vi "MSScript_Format_IonGate.vi"(9 "ValueArray":string[](array[string]), 10 "TagArray":string[](array[string]), 11 "MSScript in":refnum<class "MSScript.lvclass">) -> (0 "ValueErrorArray":bool[](array[boolean]), 1 "TagErrorArray":bool[](array[boolean]), 2 "ParamErrorArray":bool[](array[boolean]), 3 "Data":variant, 4 "#ofParamError":bool)   [LabVIEW 2018, in "MSScript.lvclass"]
uses:
  MSScript.lvclass
  Ctl/MSEditorParam ionGate.ctl
  MSScript_Transform_Boolean.vi
  MSScript_Transform_Extended.vi
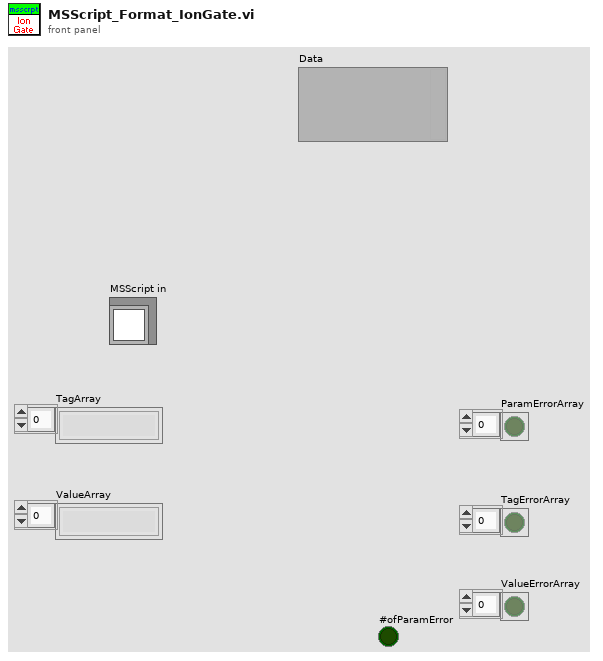
[diagram p1: front panel]
types:
  T1 = typedef "MSEditorParam ionGate.ctl" = cluster{"trialTime":ext, "TPH":ext, "enableAGC":bool}
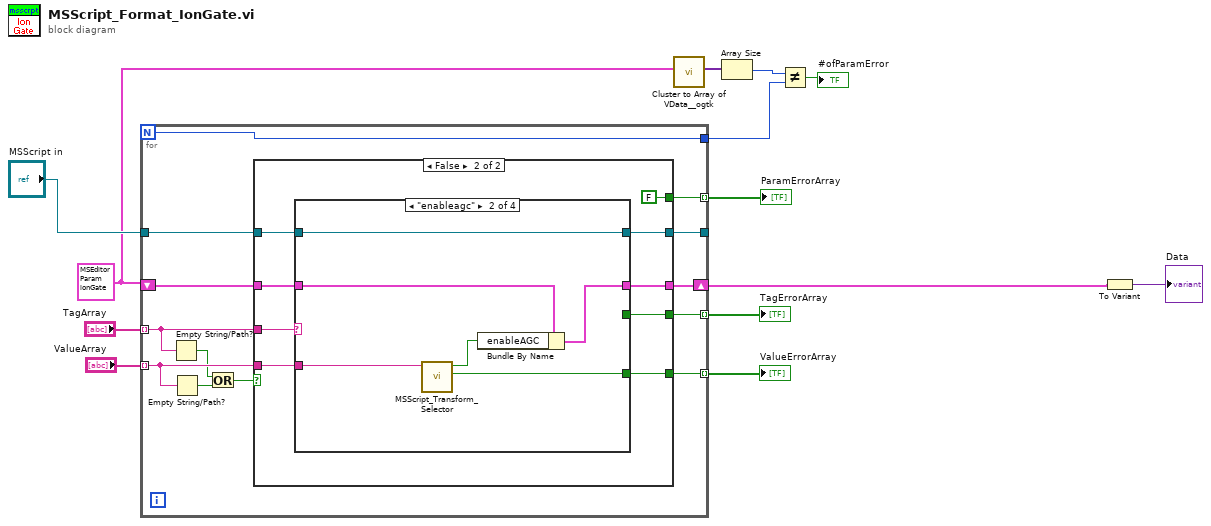
[diagram p0: block diagram]
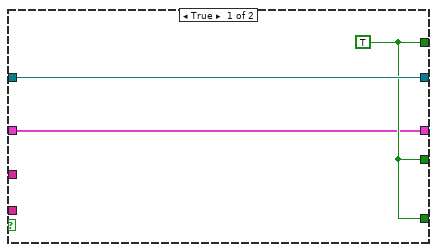
[diagram p2: hidden frame]
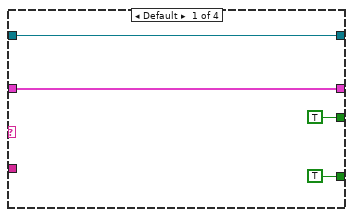
[diagram p3: hidden frame]
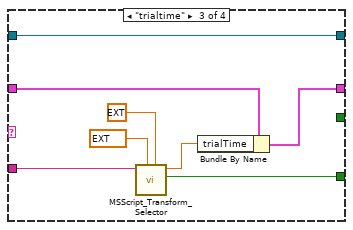
[diagram p4: hidden frame]
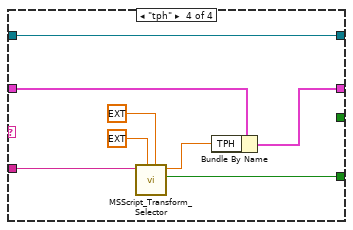
[diagram p5: hidden frame]
diagram:
  w4 = T1 {"trialTime"=0.1, "TPH"=1.0, "enableAGC"=FALSE} ("ParamValueType")
  n1 = for {
    N -> [w14]
    tunnel: "TagArray" -> [w22] mode=indexing
    tunnel: "ValueArray" -> [w21] mode=indexing
    tunnel: [w26] -> w11 mode=indexing
    tunnel: "MSScript in" -> [w25]
    tunnel: [w24] -> w10 mode=indexing
    tunnel: [w23] -> _
    tunnel: [w17] -> w9 mode=indexing
    shift-right: [w15] -> w2
    shift-left: w4 -> [w16]
    tunnel: [w14] -> w3
    n2 = Empty String/Path?(string/path=w22) -> (empty?=w19:bool)
    n3 = Empty String/Path?(string/path=w21) -> (empty?=w20:bool)
    n4 = Or(x=w19, y=w20) -> (x .or. y?=w18:bool)
    n5 = case shown="False" w18 {
      tunnel: [w28 w32] -> w26
      tunnel: w25 -> [w29 w37]
      tunnel: [w28 w33] -> w24
      tunnel: [w29 w30] -> w23
      tunnel: w22 -> [_ w35]
      tunnel: w21 -> [_ w34]
      tunnel: [w28 FALSE] -> w17
      tunnel: w16 -> [w27 w36]
      tunnel: [w27 w31] -> w15
      frame True {
        w28 = TRUE
      }
      frame False {
        n6 = case shown="\"enableagc\"" w35 {
          tunnel: [TRUE _ _ _] -> w32
          tunnel: w37 -> [w40 w46 w54 w62]
          tunnel: w34 -> [_ w47 w55 w63]
          tunnel: [TRUE ("Value Error?") w48 w56 w64] -> w33
          tunnel: [w40 w46 w54 w62] -> w30
          tunnel: w36 -> [w39 w44 w52 w60]
          tunnel: [w39 w43 w51 w59] -> w31
          frame Default {
          }
          frame "enableagc" {
            n7 = call-poly "MSScript_Transform_Selector.vi"("Check_Str"=w47) -> ("Value Error?"=w48:bool, "Value Output"=w45:bool)  [unwired: 9 in]
            n8 = Bundle By Name(cluster=w44, "enableAGC"=w45) -> (w43:T1)
          }
          frame "trialtime" {
            n9 = call-poly "MSScript_Transform_Selector.vi"("upper limit (Inf)"=ext 5.0 ("upper limit"), "lower limit (-Inf)"=ext 0.001 ("lower limit"), "Check_Str"=w55) -> ("Value Error?"=w56:bool, "Value Output"=w53:ext)  [unwired: 6 in, 1 out]
            n10 = Bundle By Name(cluster=w52, "trialTime"=w53) -> (w51:T1)
          }
          frame "tph" {
            n11 = call-poly "MSScript_Transform_Selector.vi"("upper limit (Inf)"=ext 5.0 ("upper limit"), "lower limit (-Inf)"=ext 0.0 ("lower limit"), "Check_Str"=w63) -> ("Value Error?"=w64:bool, "Value Output"=w61:ext)  [unwired: 6 in, 1 out]
            n12 = Bundle By Name(cluster=w60, "TPH"=w61) -> (w59:T1)
          }
        }
      }
    }
  }
  "TagErrorArray" <- w11
  "ValueErrorArray" <- w10
  "ParamErrorArray" <- w9
  n13 = call <userlib>:"Cluster to Array of VData__ogtk.vi"("Cluster"=w4) -> ("Array of VData"=w7:variant[])  [unwired: 9 in, 1 out]
  n14 = Array Size(array=w7) -> (size(s)=w6:i32)
  n15 = Not Equal?(x=w6, y=w3) -> (x != y?=→"#ofParamError":bool)
  n16 = To Variant(anything=w2) -> (Variant=→"Data":variant)
